vi "Configuration Window.vi"(8 "error in (no error)":errorcluster, 11 "Example Instrument in":refnum<class "Instrument.Element2.lvclass">) -> (0 "error out":errorcluster, 3 "Example Instrument out":refnum<class "Instrument.Element2.lvclass">)   [LabVIEW 2019, in "Instrument.Element2.lvclass"]
uses:
  Instrument.Element2.lvclass
  <userlib>/LevyLab/Instrument Framework/Instrument Types/VSource/Instrument.VSource.lvclass
panel:
  in  "Example Setting 3":string
  in  "Example Setting 2":dbl
  in  "Example Setting 1":dbl
  in  "Cancel":bool
  in  "OK":bool
  # "confirm or make changes:"
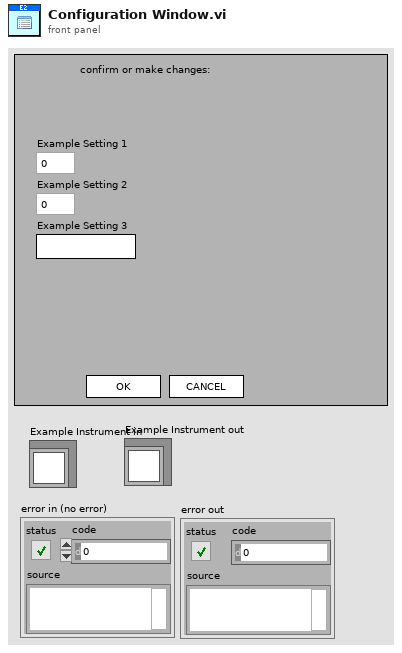
[diagram p1: front panel]
types:
  T1 = enum32{"Invalid", "Standard", "Closed", "Hidden", "Minimized", "Maximized"}
  T2 = enum32{"invalid app kind", "Development System", "Run Time System", "Student Edition", "Embedded LabVIEW", "Evaluation", "Custom"}
  T3 = typedef "Instrument.Element2.lvclass/Instrument.Element2.Configuration--Cluster.ctl" = cluster{"Example Setting 1":dbl, "Example Setting 2":dbl, "Example Setting 3":string}
  T4 = cluster{"Core":cluster{"Current VI Reference":refnum<vi>, "Close Panel on Exit?":bool}, "Configuration":T3}
  T5 = cluster{"Current VI Reference":refnum<vi>, "Close Panel on Exit?":bool}
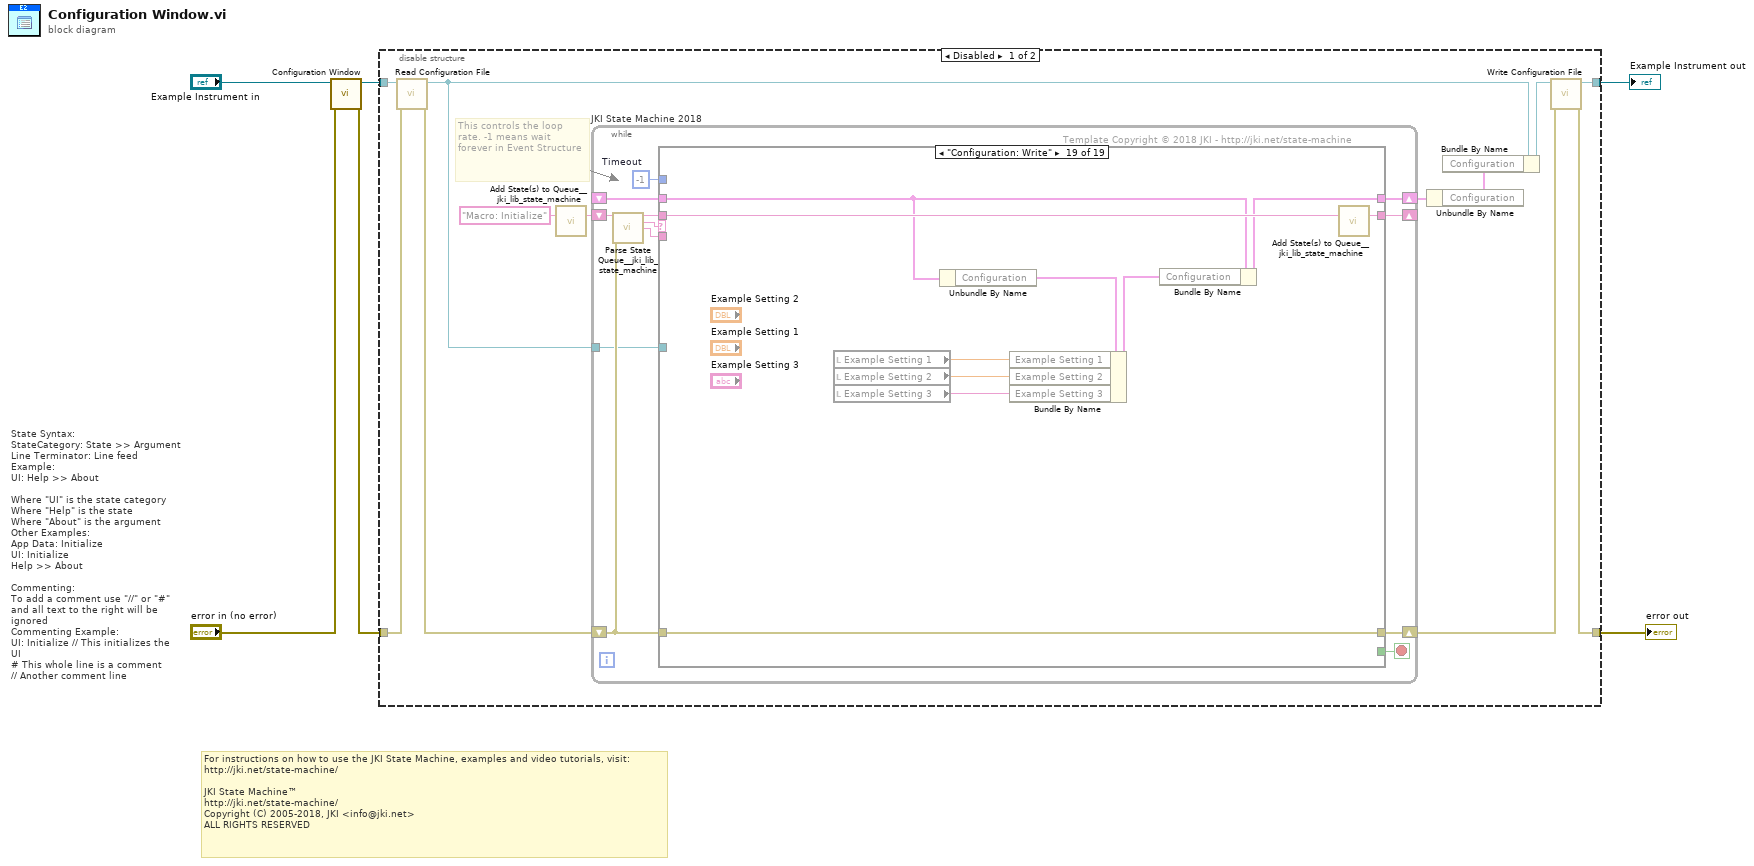
[diagram p0: block diagram]
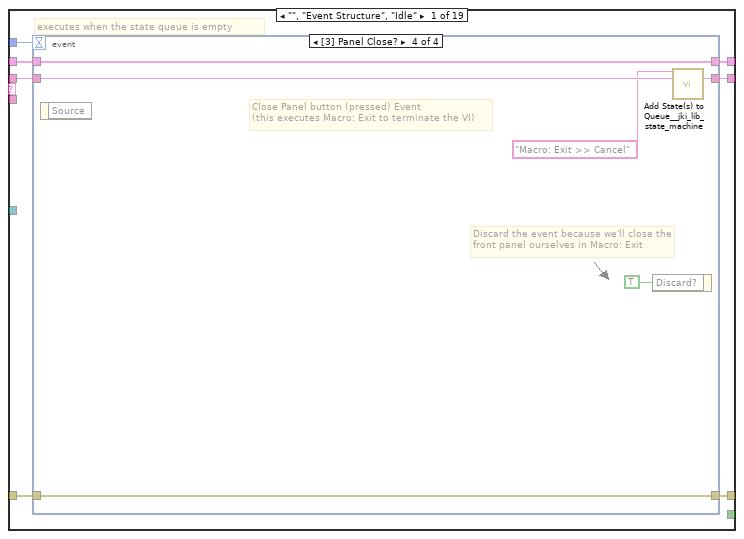
[diagram p2: hidden frame]
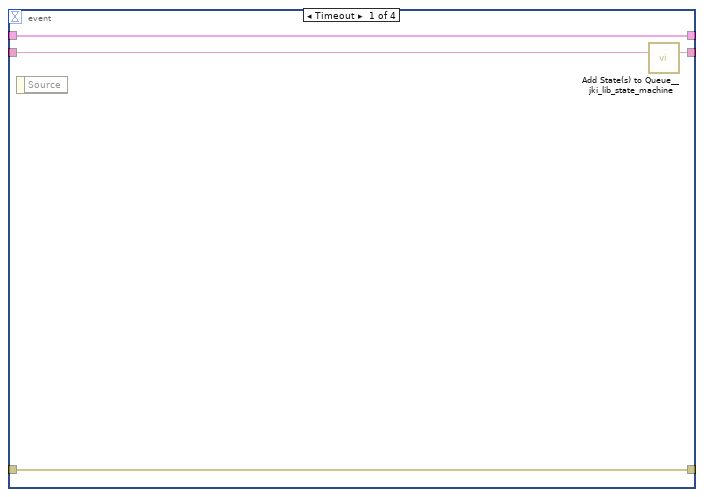
[diagram p3: hidden frame]
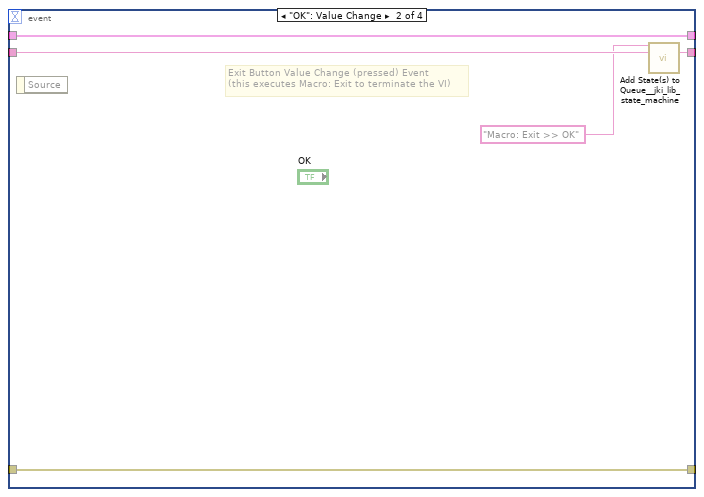
[diagram p4: hidden frame]
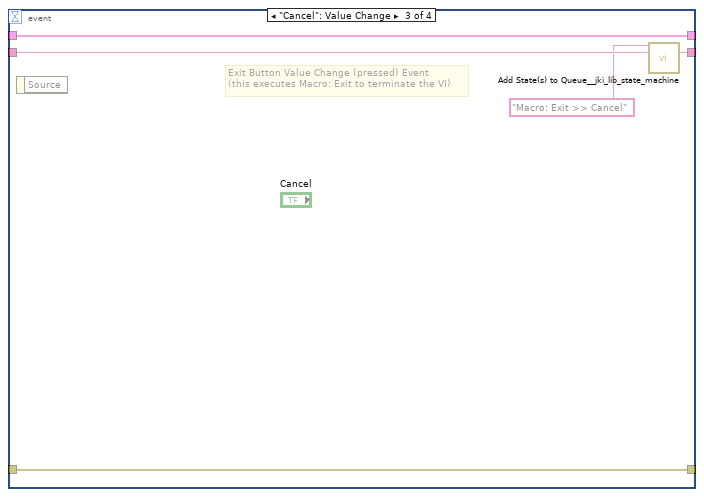
[diagram p5: hidden frame]
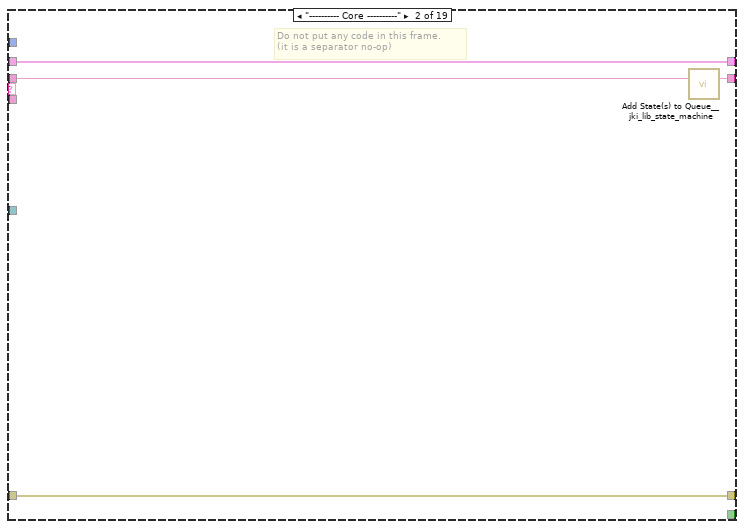
[diagram p6: hidden frame]
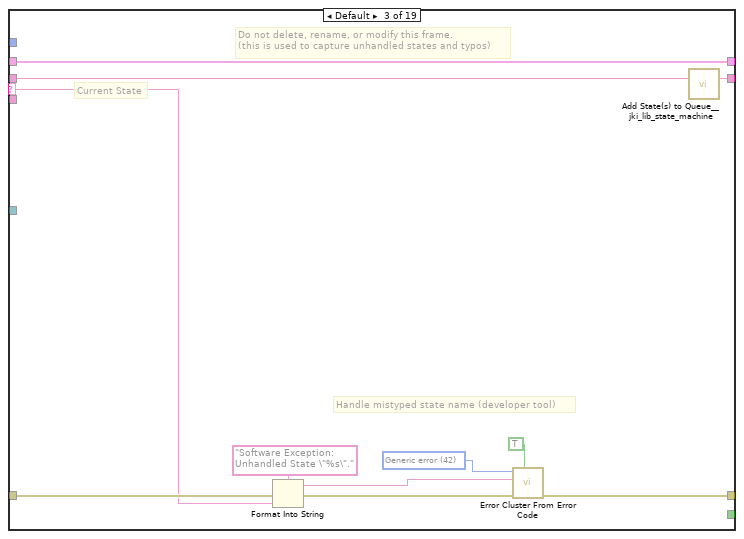
[diagram p7: hidden frame]
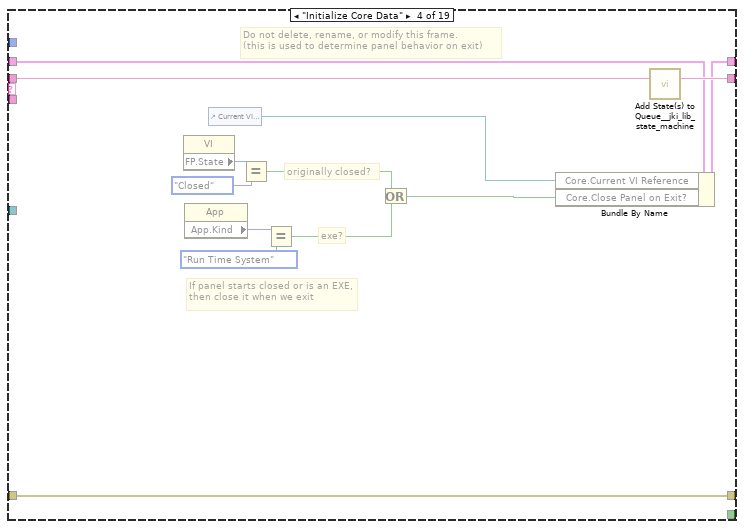
[diagram p8: hidden frame]
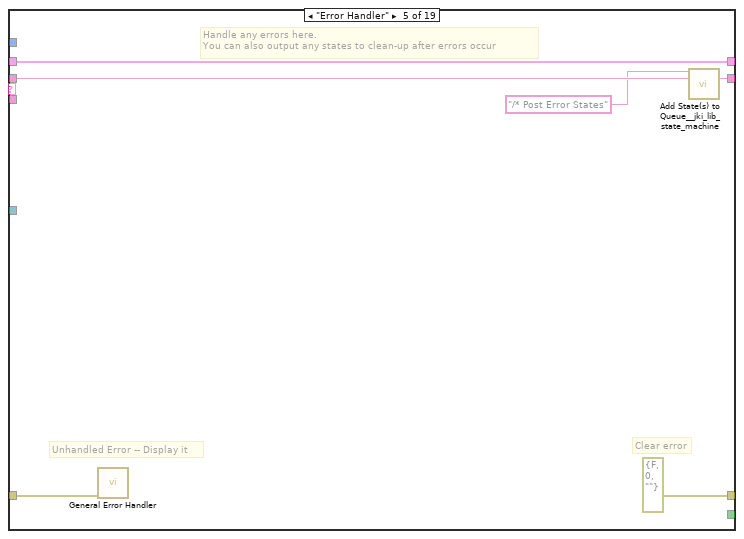
[diagram p9: hidden frame]
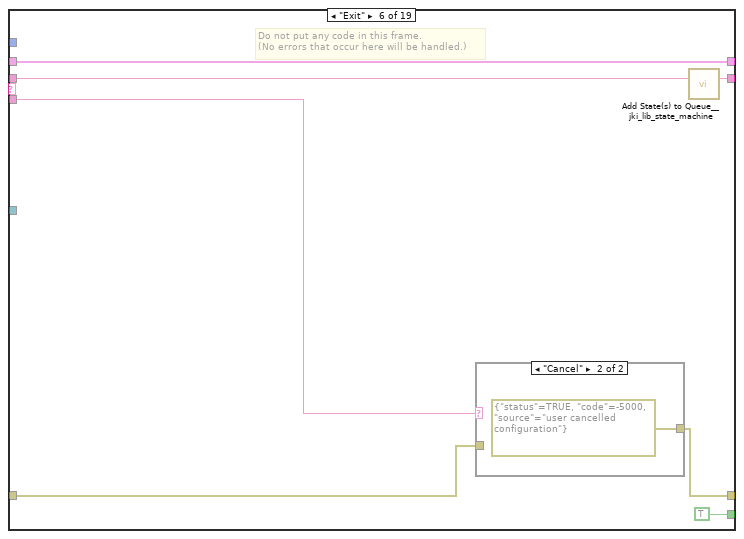
[diagram p10: hidden frame]
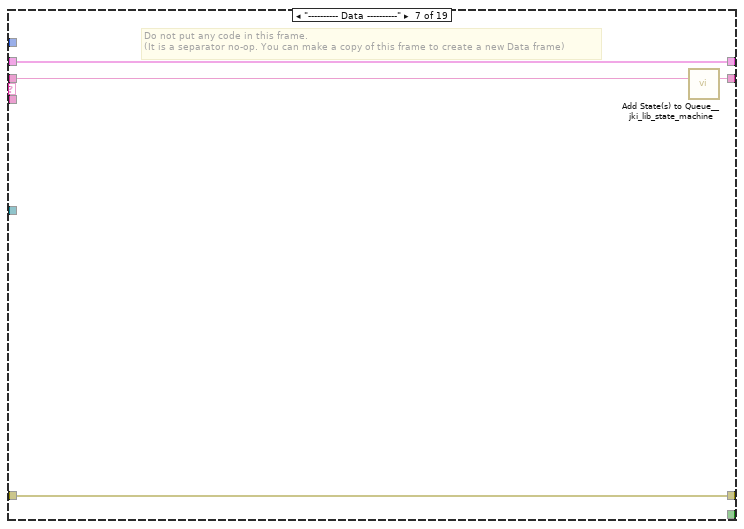
[diagram p12: hidden frame]
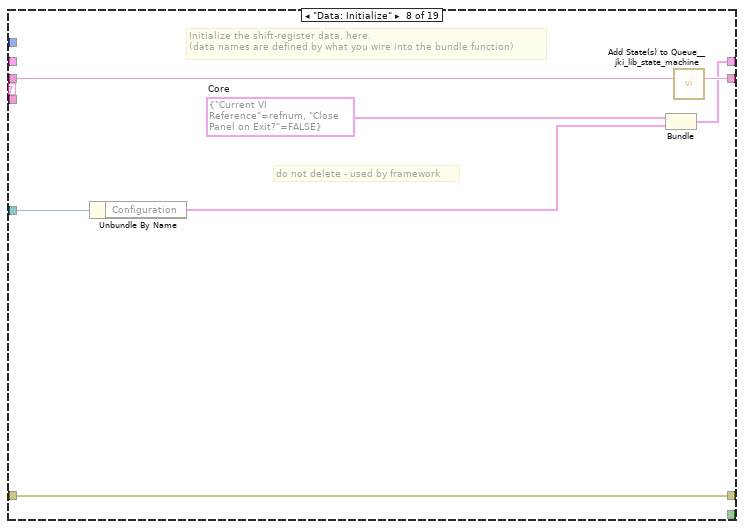
[diagram p13: hidden frame]
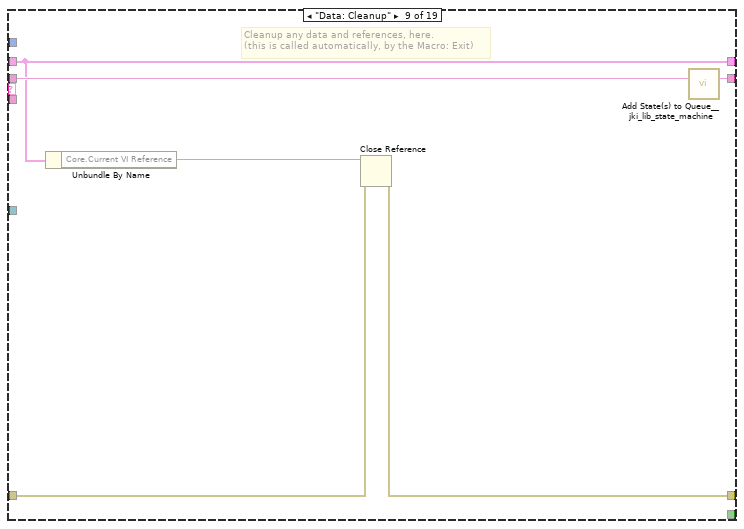
[diagram p14: hidden frame]
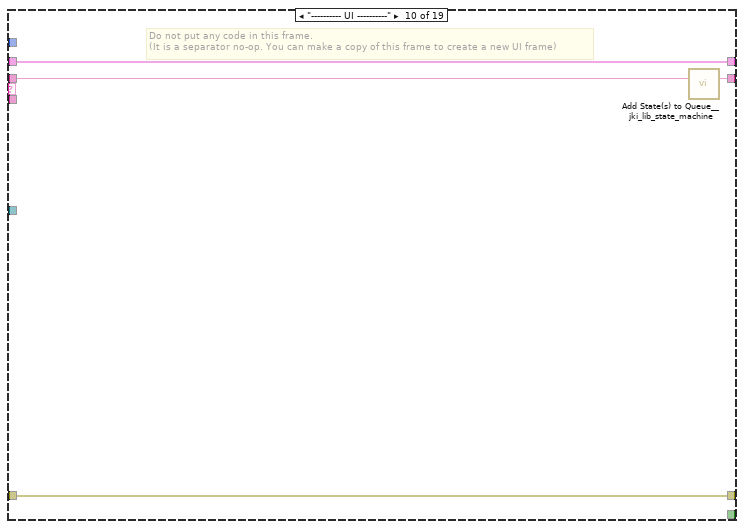
[diagram p15: hidden frame]
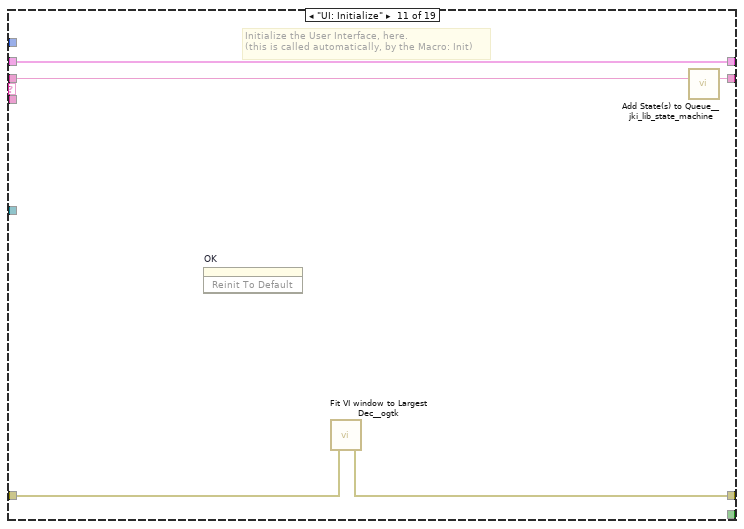
[diagram p16: hidden frame]
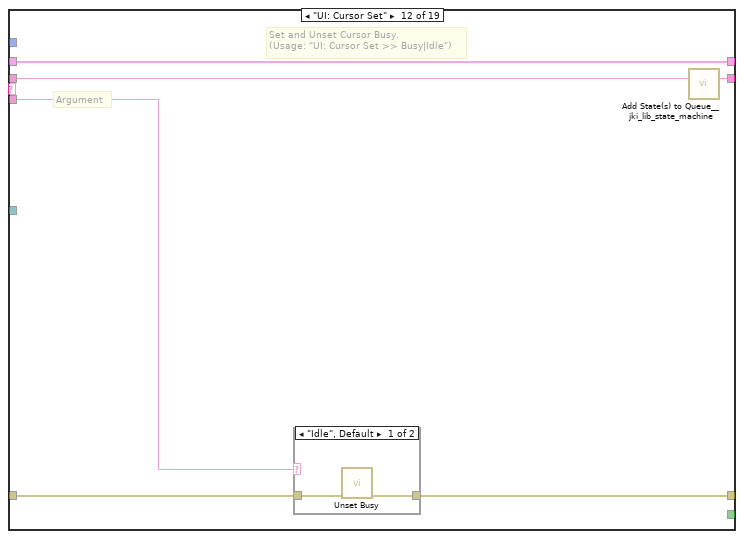
[diagram p17: hidden frame]
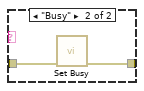
[diagram p18: hidden frame]
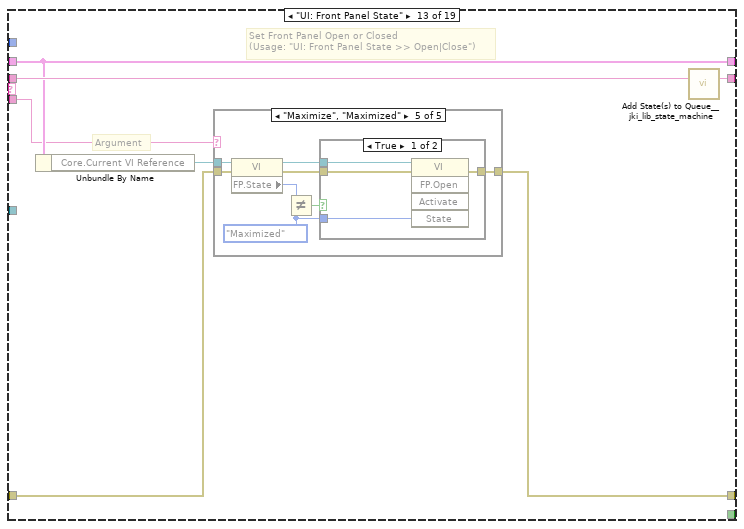
[diagram p19: hidden frame]
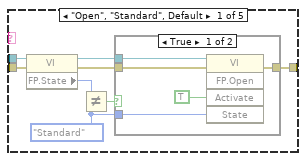
[diagram p20: hidden frame]
diagram:
  # "For instructions on how to use the JKI State Machine, examples and video tutorials, visit:\nhttp://jki.net/state-machine/\n\nJKI State Machine™\nhttp://jki.net/state-machine/\nCopyright (C) 2005-2018, JKI <info@jki.net>\nALL RIGHTS RESERVED"
  # "State Syntax:\nStateCategory: State >> Argument\nLine Terminator: Line feed\nExample:\nUI: Help >> About\n\nWhere \"UI\" is the state category\nWhere \"Help\" is the state\nWhere \"About\" is the argument\nOther Examples:\nApp Data: Initialize\nUI: Initialize\nHelp >> About\n\nCommenting:\nTo add a comment use \"//\" or \"#\" and all text to the right will be ignored\nCommenting Example:\nUI: Initialize // This initializes the UI\n# This whole line is a comment\n// Another comment line"
  n1 = call-parent "Configuration Window.vi"("error in (no error)"="error in (no error)", "Instrument"="Example Instrument in") -> ("error out"=w1:errorcluster, "Instrument out"=w3:refnum<class "Instrument.Element2.lvclass">)  [unwired: 8 in]
  n2 = disable-structure shown="Disabled" {
    disable-tunnel: [w12 w255] -> w6
    disable-tunnel: [w10 w256] -> w5
    disable-tunnel: w3 -> [w8 w255]
    disable-tunnel: w1 -> [w7 w256]
    frame Disabled {
      # "This controls the loop rate. -1 means wait forever in Event Structure"
      n3 = call-dynamic "Read Configuration File.vi"("error in (no error)"=w7, "Example Instrument in"=w8) -> ("error out"=w9:errorcluster, "Example Instrument out"=w14:refnum<class "Instrument.Element2.lvclass">)  [unwired: 8 in]
      n4 = call <vilib>:"Add State(s) to Queue__jki_lib_state_machine.vi"("State(s) in (\"\")"="Macro: Initialize") -> ("States Out"=w18:string)  [unwired: 14 in]
      n5 = while "JKI State Machine 2018" {
        shift-right: [w23] -> w16
        shift-left: _ -> [w22]
        shift-right: [w26] -> w11
        shift-left: w9 -> [w20]
        shift-right: [w25] -> _
        shift-left: w18 -> [w27]
        tunnel: w14 -> [w19]
        stop <- w24 stop-if-true
        w21 = -1  # Timeout
        # "Template Copyright © 2018 JKI - http://jki.net/state-machine"
        n6 = call <vilib>:"Parse State Queue__jki_lib_state_machine.vi"("State Queue"=w27, "Error In (no error)"=w20) -> ("Remaining States"=w29:string, "Current State"=w30:string, "Arguments"=w28:string)  [unwired: 11 in]
        n7 = case shown="\"Configuration: Write\"" w30 {
          selector: w30 -> [_ _ w62 _ _ _ _ _ _ _ _ _ _ _ _ _ _ _ _]
          tunnel: w29 -> [w37 w61 w66 w85 w91 w98 w104 w111 w117 w121 w126 w132 w143 w212 w217 w232 w236 w244 w254]
          tunnel: w28 -> [_ _ _ _ _ w94 _ _ _ _ _ w127 w137 _ _ w221 _ _ _]
          tunnel: w22 -> [w35 w58 w64 w78 w88 w96 w101 _ w112 w118 w124 w130 w139 w209 w214 w229 w233 w238 w246]
          tunnel: [w34 w59 w68 w82 errorcluster {"status"=FALSE, "code"=0, "source"=""} ("error out") w92 w102 w107 w113 w119 w122 w128 w140 w210 w215 w230 w234 w242 w252] -> w26
          tunnel: w20 -> [w33 w59 w67 w82 w87 w93 w102 w107 w114 w119 w123 w129 w141 w210 w215 w230 w234 w242 w252]
          tunnel: [w36 w60 w65 w84 w90 w97 w103 w110 w116 w120 w125 w131 w142 w211 w216 w231 w235 w243 w253] -> w25
          tunnel: [_ _ _ _ _ TRUE _ _ _ _ _ _ _ _ _ _ _ _ _] -> w24
          tunnel: [w32 w58 w64 w83 w88 w96 w101 w109 w112 w118 w124 w130 w139 w209 w214 w229 w233 w238 w245] -> w23
          tunnel: w21 -> [w31 _ _ _ _ _ _ _ _ _ _ _ _ _ _ _ _ _ _]
          tunnel: w19 -> [_ _ _ _ _ _ _ w106 _ _ _ _ _ _ _ _ _ _ _]
          frame "", "Event Structure", "Idle" {
            # "executes when the state queue is empty"
            n8 = event shown="[3] Panel Close?" {
              selector: _ -> [_ _ _ _]
              dyn-events: _ -> [_ _ _ _]
              timeout: w31 -> [_ _ _ _]
              tunnel: w37 -> [w41 w46 w51 w57]
              tunnel: [w40 w45 w50 w56] -> w36
              tunnel: w35 -> [w38 w43 w48 w54]
              tunnel: [w39 w44 w49 w55] -> w34
              tunnel: w33 -> [w39 w44 w49 w55]
              tunnel: [w38 w43 w48 w54] -> w32
              event Timeout {
                n9 = event-data() -> ()  [unwired: 1 in, 1 out]
                n10 = call <vilib>:"Add State(s) to Queue__jki_lib_state_machine.vi"("State(s) in (\"\")"=w41) -> ("States Out"=w40:string)  [unwired: 14 in]
              }
              event "OK": Value Change {
                # "Exit Button Value Change (pressed) Event\n(this executes Macro: Exit to terminate the VI)"
                n11 = event-data() -> ()  [unwired: 1 in, 1 out]
                n12 = call <vilib>:"Add State(s) to Queue__jki_lib_state_machine.vi"("State(s) in Front (\"\")"="Macro: Exit >> OK", "State(s) in (\"\")"=w46) -> ("States Out"=w45:string)  [unwired: 13 in]
              }
              event "Cancel": Value Change {
                # "Exit Button Value Change (pressed) Event\n(this executes Macro: Exit to terminate the VI)"
                n13 = event-data() -> ()  [unwired: 1 in, 1 out]
                n14 = call <vilib>:"Add State(s) to Queue__jki_lib_state_machine.vi"("State(s) in Front (\"\")"="Macro: Exit >> Cancel", "State(s) in (\"\")"=w51) -> ("States Out"=w50:string)  [unwired: 13 in]
              }
              event Panel Close? {
                # "Discard the event because we'll close the front panel ourselves in Macro: Exit"
                # "Close Panel button (pressed) Event\n(this executes Macro: Exit to terminate the VI)"
                n15 = event-data() -> ()  [unwired: 1 in, 1 out]
                n16 = event-data("Discard?"=TRUE) -> ()  [unwired: 1 in, 1 out]
                n17 = call <vilib>:"Add State(s) to Queue__jki_lib_state_machine.vi"("State(s) in Front (\"\")"="Macro: Exit >> Cancel", "State(s) in (\"\")"=w57) -> ("States Out"=w56:string)  [unwired: 13 in]
              }
            }
          }
          frame "---------- Core ----------" {
            # "Do not put any code in this frame.\n(it is a separator no-op)"
            n18 = call <vilib>:"Add State(s) to Queue__jki_lib_state_machine.vi"("State(s) in (\"\")"=w61) -> ("States Out"=w60:string)  [unwired: 14 in]
          }
          frame Default {
            w71 = 42 items=["No error", "Argument error", "Memory is full", "Out of zone", "End of file", "File already open", "Generic file I/O error", "File not found", "File permission error", "Disk is full", "Duplicate path", "Too many files open", "System feature not enabled", "Resource file not found", "Cannot add resource", "Resource not found", "Image not found", "Image memory error", "Pen does not exist", "Config type invalid", "Config token not found", "Config parse error", "Config memory error", "Bad external code format", "Bad external code offset", "External code not present", "Null window", "Destroy window error", "Null menu", "Print aborted", "Bad print record", "Print driver error", "Windows error during printing", "Memory error during printing", "Print dialog error", "Generic print error", "Invalid device refnum", "Device not found", "Device parameter error", "Device unit error", "Cannot open device", "Device call aborted", "Generic error", "Cancelled by user", "Object ID too low", "Object ID too high", "Object not in heap", "Unknown heap", "Unknown object (invalid DefProc)", "Unknown object (DefProc not in table)", "Message out of range", "Invalid (null) method", "Unknown message", "Manager call not supported", "Bad address", "Network operation in progress", "Network operation timed out", "Connection is busy", "Network attribute not supported", "Network error", "Address in use", "System out of memory", "Connection aborted", "Connection refused", "Not connected", "Already connected", "Connection closed", "Initialization error (interapplication manager)", "Bad occurrence", "Wait on unbound occurrence handler", "Occurrence queue overflow", "Datalog type conflict", "Unused", "Unrecognized type (interapplication manager)", "Memory corrupt", "Failed to make temporary DLL", "Old CIN version", "Drag socket not found", "Failed to load drop-object", "Failed to register OLE object", "Failed to release OLE object", "Format specifier type mismatch", "Unknown format specifier", "Too few format specifiers", "Too many format specifiers", "Scan failed", "Newer CIN version", "Error converting to variant", "Runtime menu error", "Password tampered", "Variant attribute not found", "Incompatible variant data type", "Event data is not available", "Event Store is not present", "Occurrence is not found", "Event Queue is not created", "Event info is not available", "Refnum passed is NULL", "Error retrieving Class GUID", "Error retrieving CoClass GUID", "Error retrieving TypeLib GUID.", "Bad built application magic bytes.", "Specific driver is different from the specific driver associated with the Logical Name.", "There is no session opened to the class driver.", "Max Error", "MAX - Error with config objects", "MAX - Error loading configuration", "MAX - Group not supported"]
            # "Current State"
            # "Do not delete, rename, or modify this frame.\n(this is used to capture unhandled states and typos)"
            # "Handle mistyped state name (developer tool)"
            n19 = Format Into String(format string="Software Exception: Unhandled State \"%s\"." ("message"), error in=w67, w62) -> (resulting string=w70:string, error out=w69:errorcluster)  [unwired: 1 in]
            n20 = call <vilib>:"Error Cluster From Error Code.vi"("show call chain? (False)"=TRUE, "error in (no error)"=w69, "error message (\"\")"=w70, "error code (0)"=w71) -> ("error out"=w68:errorcluster)  [unwired: 5 in]
            n21 = call <vilib>:"Add State(s) to Queue__jki_lib_state_machine.vi"("State(s) in (\"\")"=w66) -> ("States Out"=w65:string)  [unwired: 14 in]
          }
          frame "Initialize Core Data" {
            # "Do not delete, rename, or modify this frame.\n(this is used to determine panel behavior on exit)"
            # "originally closed?"
            # "exe?"
            # "If panel starts closed or is an EXE, then close it when we exit"
            n22 = property class="VI"() -> ("FP.State"=w75:T1)  [unwired: 2 in, 2 out]
            n23 = property class="App"() -> ("App.Kind"=w81:T2)  [unwired: 2 in, 2 out]
            n24 = control-ref of="Current VI Reference"() -> (w76:refnum<vi>)
            n25 = Equal?(x=w75, y=T1."Closed" ("Front Panel Window:State")) -> (x = y?=w73:bool)
            n26 = Equal?(x=w81, y=T2."Run Time System" ("Application:Kind")) -> (x = y?=w79:bool)
            n27 = Or(x=w73, y=w79) -> (x .or. y?=w77:bool)
            n28 = Bundle By Name(cluster=w78, "Core.Current VI Reference"=w76, "Core.Close Panel on Exit?"=w77) -> (w83:T4)
            n29 = call <vilib>:"Add State(s) to Queue__jki_lib_state_machine.vi"("State(s) in (\"\")"=w85) -> ("States Out"=w84:string)  [unwired: 14 in]
          }
          frame "Error Handler" {
            # "Unhandled Error -- Display it"
            # "Handle any errors here.\nYou can also output any states to clean-up after errors occur"
            # "Clear error"
            n30 = call <vilib>:"General Error Handler.vi"("error in (no error)"=w87) -> ()  [unwired: 10 in, 5 out]
            n31 = call <vilib>:"Add State(s) to Queue__jki_lib_state_machine.vi"("State(s) in Front (\"\")"="/* Post Error States", "State(s) in (\"\")"=w91) -> ("States Out"=w90:string)  [unwired: 13 in]
          }
          frame "Exit" {
            # "Do not put any code in this frame.\n(No errors that occur here will be handled.)"
            n32 = case shown="\"Cancel\"" w94 {
              tunnel: w93 -> [w99 _]
              tunnel: [w99 errorcluster {"status"=TRUE, "code"=-5000, "source"="user cancelled configuration"} ("error in (no error)")] -> w92
              frame "OK", Default {
              }
              frame "Cancel" {
              }
            }
            n33 = call <vilib>:"Add State(s) to Queue__jki_lib_state_machine.vi"("State(s) in (\"\")"=w98) -> ("States Out"=w97:string)  [unwired: 14 in]
          }
          frame "---------- Data ----------" {
            # "Do not put any code in this frame.\n(It is a separator no-op. You can make a copy of this frame to create a new Data frame)"
            n34 = call <vilib>:"Add State(s) to Queue__jki_lib_state_machine.vi"("State(s) in (\"\")"=w104) -> ("States Out"=w103:string)  [unwired: 14 in]
          }
          frame "Data: Initialize" {
            w108 = T5 {"Current VI Reference"=refnum, "Close Panel on Exit?"=FALSE}  # Core
            # "do not delete - used by framework"
            # "Initialize the shift-register data, here.\n(data names are defined by what you wire into the bundle function)"
            n35 = Unbundle By Name(w106) -> ("Configuration"=w105:T3)
            n36 = Bundle("Core"=w108, "Configuration"=w105) -> (w109:T4)  [unwired: 1 in]
            n37 = call <vilib>:"Add State(s) to Queue__jki_lib_state_machine.vi"("State(s) in (\"\")"=w111) -> ("States Out"=w110:string)  [unwired: 14 in]
          }
          frame "Data: Cleanup" {
            # "Cleanup any data and references, here.\n(this is called automatically, by the Macro: Exit)"
            n38 = Unbundle By Name(w112) -> ("Core.Current VI Reference"=w115:refnum<vi>)
            n39 = Close Reference(reference=w115, error in (no error)=w114) -> (error out=w113:errorcluster)
            n40 = call <vilib>:"Add State(s) to Queue__jki_lib_state_machine.vi"("State(s) in (\"\")"=w117) -> ("States Out"=w116:string)  [unwired: 14 in]
          }
          frame "---------- UI ----------" {
            # "Do not put any code in this frame.\n(It is a separator no-op. You can make a copy of this frame to create a new UI frame)"
            n41 = call <vilib>:"Add State(s) to Queue__jki_lib_state_machine.vi"("State(s) in (\"\")"=w121) -> ("States Out"=w120:string)  [unwired: 14 in]
          }
          frame "UI: Initialize" {
            # "Initialize the User Interface, here.\n(this is called automatically, by the Macro: Init)"
            n42 = invoke on="OK" class="Bool" method="Reinit To Default"() -> ()  [unwired: 3 in, 3 out]
            n43 = call <userlib>:"Fit VI window to Largest Dec__ogtk.vi"("error in (no error)"=w123) -> ("error out"=w122:errorcluster)  [unwired: 5 in, 1 out]
            n44 = call <vilib>:"Add State(s) to Queue__jki_lib_state_machine.vi"("State(s) in (\"\")"=w126) -> ("States Out"=w125:string)  [unwired: 14 in]
          }
          frame "UI: Cursor Set" {
            # "Argument"
            # "Set and Unset Cursor Busy.\n(Usage: \"UI: Cursor Set >> Busy|Idle\")"
            n45 = case shown="\"Idle\", Default" w127 {
              tunnel: w129 -> [w134 w136]
              tunnel: [w133 w135] -> w128
              frame "Idle", Default {
                n46 = call <vilib>:"Unset Busy.vi"("error in (no error)"=w134) -> ("error out"=w133:errorcluster)  [unwired: 10 in]
              }
              frame "Busy" {
                n47 = call <vilib>:"Set Busy.vi"("error in (no error)"=w136) -> ("error out"=w135:errorcluster)  [unwired: 9 in, 1 out]
              }
            }
            n48 = call <vilib>:"Add State(s) to Queue__jki_lib_state_machine.vi"("State(s) in (\"\")"=w132) -> ("States Out"=w131:string)  [unwired: 14 in]
          }
          frame "UI: Front Panel State" {
            # "Argument"
            # "Set Front Panel Open or Closed\n(Usage: \"UI: Front Panel State >> Open|Close\")"
            n49 = Unbundle By Name(w139) -> ("Core.Current VI Reference"=w138:refnum<vi>)
            n50 = case shown="\"Maximize\", \"Maximized\"" w137 {
              tunnel: w141 -> [w149 w164 w175 w188 w201]
              tunnel: [w151 w165 w177 w190 w203] -> w140
              tunnel: w138 -> [w150 w162 w176 w189 w202]
              frame "Open", "Standard", Default {
                w144 = T1."Standard" ("State")
                n51 = property class="VI"(reference=w150, error in=w149) -> (reference out=w147:refnum<vi>, error out=w148:errorcluster, "FP.State"=w146:T1)
                n52 = Not Equal?(x=w146, y=w144) -> (x != y?=w145:bool)
                n53 = case shown="True" w145 {
                  tunnel: [w155 w157] -> w151
                  tunnel: w148 -> [w154 w157]
                  tunnel: w147 -> [w153 _]
                  tunnel: w144 -> [w152 _]
                  frame True {
                    n54 = invoke class="VI" method="FP.Open"(reference=w153, error in=w154, "Activate"=TRUE, "State"=w152) -> (error out=w155:errorcluster)  [unwired: 1 in, 4 out]
                  }
                  frame False {
                  }
                }
              }
              frame "Close", "Closed" {
                n55 = property class="VI"(reference=w162, error in=w164) -> (reference out=w161:refnum<vi>, error out=w163:errorcluster, "FP.State"=w159:T1)
                n56 = Not Equal?(x=w159, y=T1."Closed" ("Front Panel Window:State")) -> (x != y?=w158:bool)
                n57 = case shown="True" w158 {
                  tunnel: [w166 w169] -> w165
                  tunnel: w163 -> [w166 w168]
                  tunnel: w161 -> [_ w167]
                  frame False {
                  }
                  frame True {
                    n58 = invoke class="VI" method="FP.Close"(reference=w167, error in=w168) -> (error out=w169:errorcluster)  [unwired: 1 in, 2 out]
                  }
                }
              }
              frame "Hidden", "Hide" {
                w170 = T1."Hidden" ("State")
                n59 = property class="VI"(reference=w176, error in=w175) -> (reference out=w173:refnum<vi>, error out=w174:errorcluster, "FP.State"=w172:T1)
                n60 = Not Equal?(x=w172, y=w170) -> (x != y?=w171:bool)
                n61 = case shown="True" w171 {
                  tunnel: [w181 w182] -> w177
                  tunnel: w174 -> [w180 w182]
                  tunnel: w173 -> [w179 _]
                  tunnel: w170 -> [w178 _]
                  frame True {
                    n62 = invoke class="VI" method="FP.Open"(reference=w179, error in=w180, "State"=w178) -> (error out=w181:errorcluster)  [unwired: 2 in, 4 out]
                  }
                  frame False {
                  }
                }
              }
              frame "Minimize", "Minimized" {
                w183 = T1."Minimized" ("State")
                n63 = property class="VI"(reference=w189, error in=w188) -> (reference out=w186:refnum<vi>, error out=w187:errorcluster, "FP.State"=w185:T1)
                n64 = Not Equal?(x=w185, y=w183) -> (x != y?=w184:bool)
                n65 = case shown="True" w184 {
                  tunnel: [w194 w195] -> w190
                  tunnel: w187 -> [w193 w195]
                  tunnel: w186 -> [w192 _]
                  tunnel: w183 -> [w191 _]
                  frame True {
                    n66 = invoke class="VI" method="FP.Open"(reference=w192, error in=w193, "State"=w191) -> (error out=w194:errorcluster)  [unwired: 2 in, 4 out]
                  }
                  frame False {
                  }
                }
              }
              frame "Maximize", "Maximized" {
                w196 = T1."Maximized" ("State")
                n67 = property class="VI"(reference=w202, error in=w201) -> (reference out=w199:refnum<vi>, error out=w200:errorcluster, "FP.State"=w198:T1)
                n68 = Not Equal?(x=w198, y=w196) -> (x != y?=w197:bool)
                n69 = case shown="True" w197 {
                  tunnel: [w207 w208] -> w203
                  tunnel: w200 -> [w206 w208]
                  tunnel: w199 -> [w205 _]
                  tunnel: w196 -> [w204 _]
                  frame True {
                    n70 = invoke class="VI" method="FP.Open"(reference=w205, error in=w206, "State"=w204) -> (error out=w207:errorcluster)  [unwired: 2 in, 4 out]
                  }
                  frame False {
                  }
                }
              }
            }
            n71 = call <vilib>:"Add State(s) to Queue__jki_lib_state_machine.vi"("State(s) in (\"\")"=w143) -> ("States Out"=w142:string)  [unwired: 14 in]
          }
          frame "---------- Macro ----------" {
            # "Do not put any code in this frame.\n(It is a separator no-op. You can make a copy of this frame to create a new Macro frame)"
            n72 = call <vilib>:"Add State(s) to Queue__jki_lib_state_machine.vi"("State(s) in (\"\")"=w212) -> ("States Out"=w211:string)  [unwired: 14 in]
          }
          frame "Macro: Initialize" {
            w213 = "Data: Initialize\nInitialize Core Data\nUI: Initialize\nUI: Front Panel State >> Open\nConfiguration: Read"  # Data: Initialize Initialize Core Data UI: Initialize UI: Front Panel State >> Open Configuration: Read
            # "Initialization Macro\n(This is called once, when the VI starts)"
            n73 = call <vilib>:"Add State(s) to Queue__jki_lib_state_machine.vi"("State(s) in Front (\"\")"=w213, "State(s) in (\"\")"=w217) -> ("States Out"=w216:string)  [unwired: 13 in]
          }
          frame "Macro: Exit" {
            # "Exit Macro\n(This is called once, when the VI exits)"
            n74 = Unbundle By Name(w229) -> ("Core.Close Panel on Exit?"=w228:bool)
            n75 = call <vilib>:"Build State String with Arguments__JKI_lib_State_Machine.vi"("Arguments (\"\")"=w221, "State"="Exit") -> ("State with Arguments"=w219:string)  [unwired: 4 in]
            n76 = Select(t="UI: Front Panel State >> Close", s=w228, f="") -> (s? t:f=w225:string)
            n77 = call <vilib>:"Add State(s) to Queue__jki_lib_state_machine.vi"("State(s) in Front (\"\")"="Data: Cleanup", "State(s) at Back (\"\")"=w219) -> ("States Out"=w218:string)  [unwired: 13 in]
            n78 = call <vilib>:"Add State(s) to Queue__jki_lib_state_machine.vi"("State(s) in Front (\"\")"="Configuration: Write", "State(s) in (\"\")"=w225, "State(s) at Back (\"\")"=w218) -> ("States Out"=w224:string)  [unwired: 12 in]
            n79 = call <vilib>:"Add State(s) to Queue__jki_lib_state_machine.vi"("State(s) in Front (\"\")"=w224, "State(s) in (\"\")"=w232) -> ("States Out"=w231:string)  [unwired: 13 in]
          }
          frame "---------- Configuration ----------" {
            # "Template Separator\n(You can make a copy of, or modify, this frame)"
            n80 = call <vilib>:"Add State(s) to Queue__jki_lib_state_machine.vi"("State(s) in (\"\")"=w236) -> ("States Out"=w235:string)  [unwired: 14 in]
          }
          frame "Configuration: Read" {
            # "Your code here.\n(You can make a copy of, or modify, this frame)"
            n81 = Unbundle By Name(w238) -> ("Configuration"=w237:T3)
            n82 = Unbundle By Name(w237) -> ("Example Setting 1"=w241:dbl, "Example Setting 2"=w240:dbl, "Example Setting 3"=w239:string)
            n83 = local write "Example Setting 2"(w240) -> ()
            n84 = local write "Example Setting 1"(w241) -> ()
            n85 = local write "Example Setting 3"(w239) -> ()
            n86 = call <vilib>:"Add State(s) to Queue__jki_lib_state_machine.vi"("State(s) in (\"\")"=w244) -> ("States Out"=w243:string)  [unwired: 14 in]
          }
          frame "Configuration: Write" {
            n87 = local read "Example Setting 1"() -> (w251:dbl)
            n88 = local read "Example Setting 2"() -> (w248:dbl)
            n89 = local read "Example Setting 3"() -> (w249:string)
            n90 = Unbundle By Name(w246) -> ("Configuration"=w250:T3)
            n91 = Bundle By Name(cluster=w250, "Example Setting 1"=w251, "Example Setting 2"=w248, "Example Setting 3"=w249) -> (w247:T3)
            n92 = Bundle By Name(cluster=w246, "Configuration"=w247) -> (w245:T4)
            n93 = call <vilib>:"Add State(s) to Queue__jki_lib_state_machine.vi"("State(s) in (\"\")"=w254) -> ("States Out"=w253:string)  [unwired: 14 in]
          }
        }
      }
      n94 = Unbundle By Name(w16) -> ("Configuration"=w15:T3)
      n95 = Bundle By Name(cluster=w14, "Configuration"=w15) -> (w13:refnum<class "Instrument.Element2.lvclass">)
      n96 = call-dynamic "Write Configuration File.vi"("error in (no error)"=w11, "Example Instrument in"=w13) -> ("error out"=w10:errorcluster, "Example Instrument out"=w12:refnum<class "Instrument.Element2.lvclass">)  [unwired: 8 in]
    }
    frame Enabled {
    }
  }
  "error out" <- w5
  "Example Instrument out" <- w6
